vi "Gripper.vi"() -> ()   [LabVIEW 2013]
uses:
  ROS/Code/SubVIs/BaxterButtons.ctl
  ROS/Code/SubVIs/BaxterSide.ctl
panel:
  in  "Calibrate":bool
  in  "Close":bool
  in  "Open":bool
  in  "Functions":i32[](listbox)=[2, 4]
  out "Gripper State":bool=TRUE
  in  "stop":bool
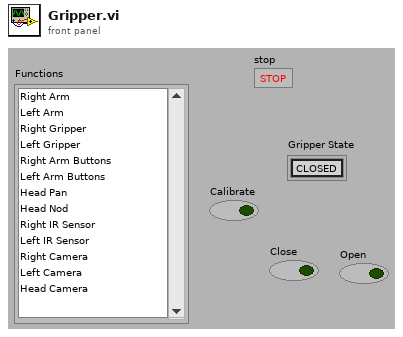
[diagram p1: front panel]
types:
  T1 = typedef "BaxterButtons.ctl" = u16
  T2 = typedef "BaxterSide.ctl" = enum16{"left", "right"}
  T3 = cluster{"Cancel":bool, "OK":bool, "Show":bool, "Wheel":u8}
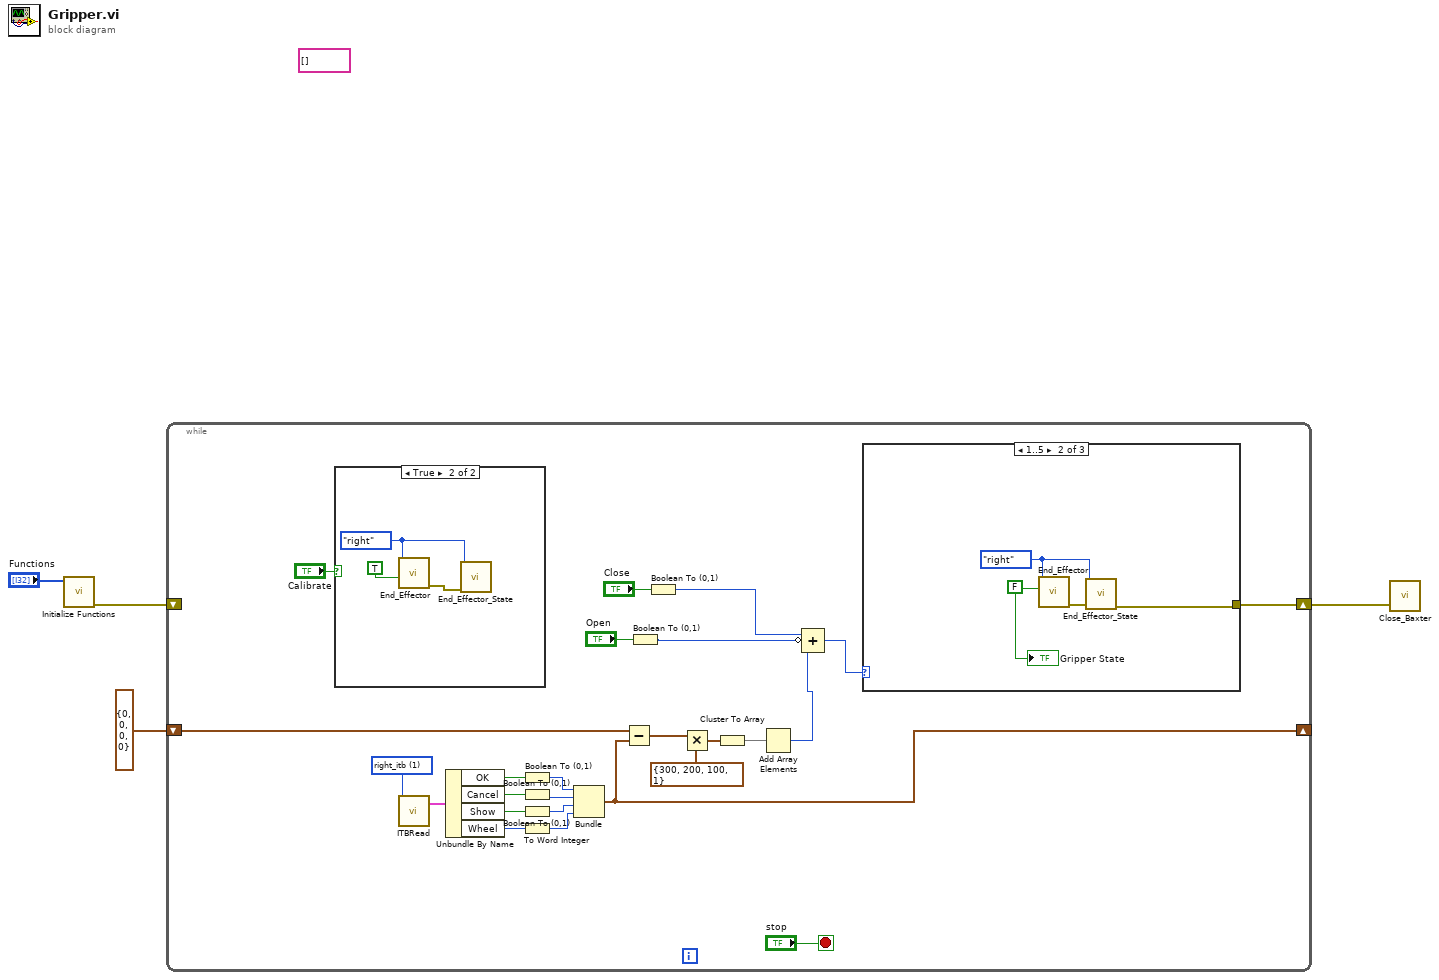
[diagram p0: block diagram]
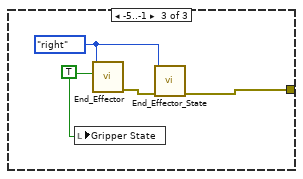
[diagram p4: hidden frame]
diagram:
  (unwired) string[] [] ("Item Names")
  n1 = call "Initialize Functions.vi"("Functions"="Functions") -> ("error out"=w4:errorcluster)  [unwired: 10 in]
  n2 = while {
    shift-right: [w28] -> _
    shift-left: cluster{i16, i16, i16, i16} {0, 0, 0, 0} -> [w29]
    shift-right: [w27] -> w2
    shift-left: w4 -> [_]
    stop <- "stop" stop-if-true
    w25 = T1 1 items=["left_itb", "right_itb", "torso_left_itb", "torso_right_itb"] ("Component")
    n3 = case shown="True" "Calibrate" {
      frame False {
      }
      frame True {
        w31 = BaxterSide."right" ("Side")
        n4 = call "End_Effector.vi"("Calibrate"=TRUE, "Side"=w31) -> ("error out"=w32:errorcluster)  [unwired: 6 in]
        n5 = call "End_Effector_State.vi"("error in"=w32, "Side"=w31) -> ()  [unwired: 5 in, 2 out]
      }
    }
    n6 = call "ITBRead.vi"("Component"=w25) -> ("ITB"=w24:T3)  [unwired: 2 in, 1 out]
    n7 = Unbundle By Name(w24) -> ("OK"=w23:bool, "Cancel"=w22:bool, "Show"=w21:bool, "Wheel"=w19:u8)
    n8 = Boolean To (0,1)(Boolean=w23) -> (0, 1=w20:i16)
    n9 = Boolean To (0,1)(Boolean=w22) -> (0, 1=w17:i16)
    n10 = Boolean To (0,1)(Boolean=w21) -> (0, 1=w18:i16)
    n11 = To Word Integer(number=w19) -> (16bit integer=w16:i16)
    n12 = Bundle(w20, w17, w18, w16) -> (w28:cluster{i16, i16, i16, i16})  [unwired: 1 in]
    n13 = Subtract(x=w29, y=w28) -> (x-y=w15:cluster{i16, i16, i16, i16})
    n14 = Boolean To (0,1)(Boolean="Open") -> (0, 1=w10:i16)
    n15 = Boolean To (0,1)(Boolean="Close") -> (0, 1=w8:i16)
    n16 = Multiply(x=w15, y=cluster{i16, i16, i16, i16} {300, 200, 100, 1}) -> (x*y=w13:cluster{i16, i16, i16, i16})
    n17 = Cluster To Array(cluster=w13) -> (array=w12:i16[])
    n18 = Add Array Elements(numeric array=w12) -> (sum=w7:i16)
    n19 = Compound Arithmetic op=ADD(w8, invert w10, w7) -> (w6:i16)
    n20 = case shown="1..5" w6 {
      tunnel: [_ w35 w38] -> w27
      frame Default {
      }
      frame 1..5 {
        w34 = BaxterSide."right" ("Side")
        w33 = FALSE ("Calibrate")
        n21 = call "End_Effector.vi"("Open"=w33, "Side"=w34) -> ("error out"=w36:errorcluster)  [unwired: 6 in]
        n22 = call "End_Effector_State.vi"("error in"=w36, "Side"=w34) -> ("error out"=w35:errorcluster)  [unwired: 5 in, 1 out]
        "Gripper State" <- w33
      }
      frame -5..-1 {
        w37 = BaxterSide."right" ("Side")
        w40 = TRUE ("Calibrate")
        n23 = local write "Gripper State"(w40) -> ()
        n24 = call "End_Effector.vi"("Open"=w40, "Side"=w37) -> ("error out"=w39:errorcluster)  [unwired: 6 in]
        n25 = call "End_Effector_State.vi"("error in"=w39, "Side"=w37) -> ("error out"=w38:errorcluster)  [unwired: 5 in, 1 out]
      }
    }
  }
  n26 = call "Close_Baxter.vi"("error in"=w2) -> ()  [unwired: 3 in, 1 out]
